vi "ex_Change Control Name.vi"(4 "error in (no error)":errorcluster, 5 "New Name":string, 6 "Old Name":string, 7 "VI refnum":refnum<vi>) -> (0 "error out":errorcluster, 2 "Array":string[](array[string]), 3 "Ctl refnum out":refnum<vi>)   [LabVIEW 2020]
doc: "Changes the label and the caption for a control specified by the control refnum on the VI specified by the VI refnum."
panel:
  in  "Ctl refnum":refnum<vi>
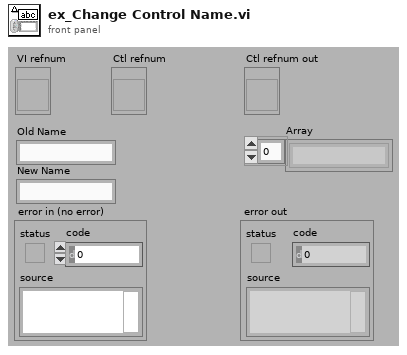
[diagram p1: front panel]
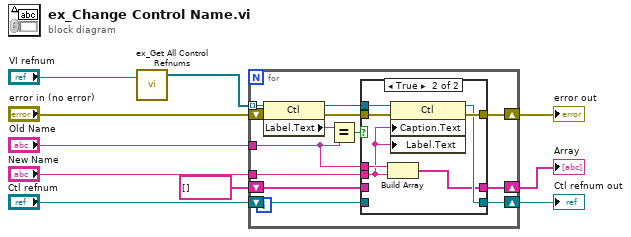
[diagram p0: block diagram]
diagram:
  n1 = call <vilib>:"ex_Get All Control Refnums.vi"("viref Express VI"="VI refnum") -> ("All Controls[]"=w2:refnum<vi>[])  [unwired: 2 in, 1 out]
  n2 = for {
    tunnel: w2 -> [w23] mode=indexing
    tunnel: "Old Name" -> [w13]
    tunnel: "New Name" -> [w20]
    shift-right: [w17] -> w4
    shift-left: "error in (no error)" -> [w16]
    shift-right: [w15] -> w7
    shift-left: "Ctl refnum" -> [w14]
    shift-right: [w12] -> w6
    shift-left: string[] [] -> [w11]
    n3 = property class="Ctl"(reference=w23, error in=w16) -> (reference out=w21:refnum<vi>, error out=w18:errorcluster, "Label.Text"=w22:string)
    n4 = Equal?(x=w22, y=w13) -> (x = y?=w19:bool)
    n5 = case shown="True" w19 {
      tunnel: w21 -> [_ w33]
      tunnel: w20 -> [_ w28]
      tunnel: w18 -> [w26 w32]
      tunnel: [w26 w31] -> w17
      tunnel: [w25 w30] -> w15
      tunnel: w14 -> [w25 _]
      tunnel: w13 -> [_ w29]
      tunnel: [w24 w27] -> w12
      tunnel: w11 -> [w24 _]
      frame False {
      }
      frame True {
        n6 = Build Array(w29, w28) -> (w27:string[])
        n7 = property class="Ctl"(reference=w33, error in=w32, "Caption.Text"=w28, "Label.Text"=w28) -> (reference out=w30:refnum<vi>, error out=w31:errorcluster)
      }
    }
  }
  "error out" <- w4
  "Ctl refnum out" <- w7
  "Array" <- w6
